vi "SetNeoParams.vi"(4 "Error In":errorcluster, 5 "Debug":bool=TRUE) -> (0 "ErrorOut":errorcluster, 3 "Handle":i32)   [LabVIEW 2014]
panel:
  in  "PreAmp Gain Control":string(combo)="16-bit (low noise & high well capacity)"
  out "Stat: preamp":i32
  in  "Cluster":T1={"ExposureTime"=0.1, "AOI Height"=2160, "AOI Width"=2560}
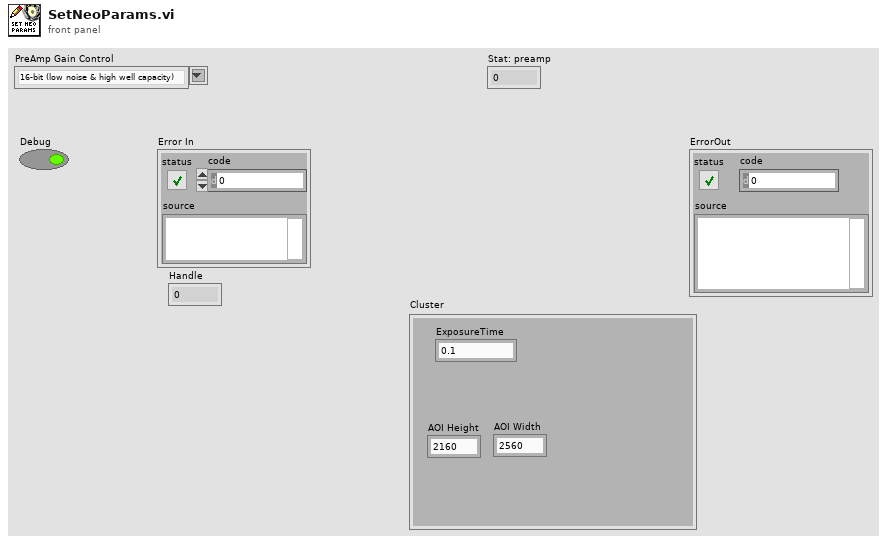
[diagram p1: front panel]
types:
  T1 = cluster{"ExposureTime":dbl, "AOI Height":i32, "AOI Width":i32}
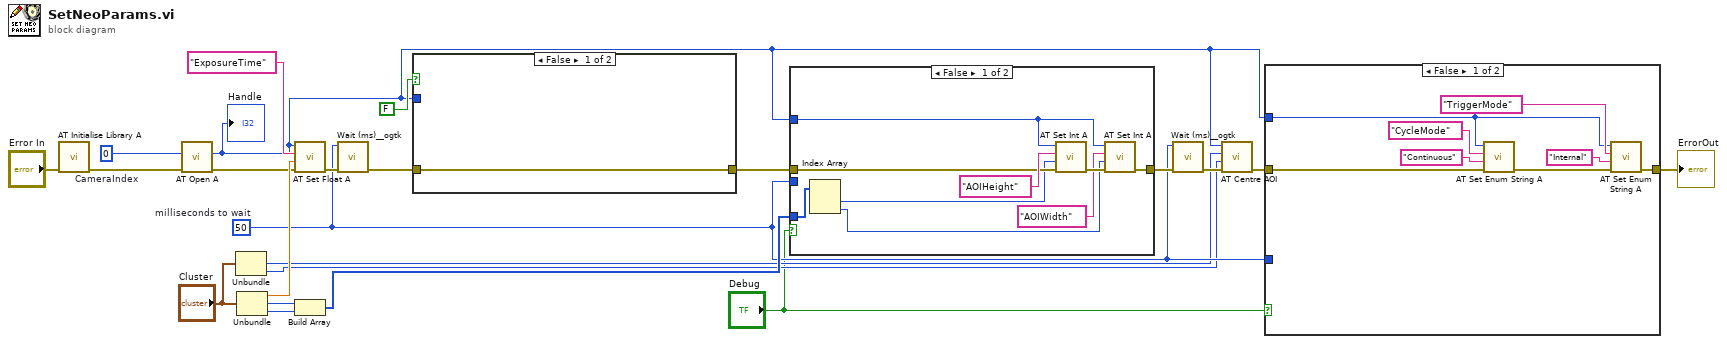
[diagram p0: block diagram]
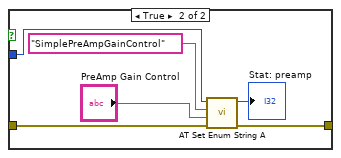
[diagram p2: hidden frame]
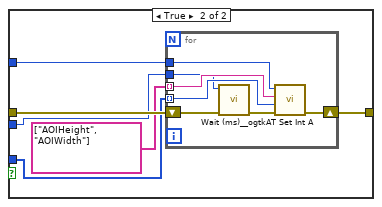
[diagram p3: hidden frame]
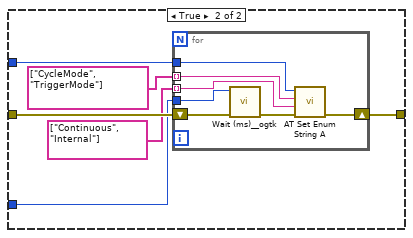
[diagram p4: hidden frame]
diagram:
  w4 = 0  # CameraIndex
  w13 = u32 50  # milliseconds to wait
  n1 = call <userlib>:"AT Initialise Library A.vi"("error in (no error)"="Error In") -> ("error out"=w5:errorcluster)  [unwired: 9 in, 1 out]
  n2 = call <userlib>:"AT Open A.vi"("error in (no error)"=w5, "CameraIndex"=w4) -> ("error out"=w3:errorcluster, "Handle"=w1:i32)  [unwired: 7 in, 1 out]
  "Handle" <- w1
  n3 = Unbundle("Cluster") -> ("AOI Height"=w10:i32, "AOI Width"=w9:i32)  [unwired: 1 out]
  n4 = Unbundle("Cluster") -> ("ExposureTime"=w20:dbl, "AOI Height"=w12:i32, "AOI Width"=w11:i32)
  n5 = call <userlib>:"AT Set Float A.vi"("error in (no error)"=w3, "Value"=w20, "Feature"="ExposureTime" ("ExposureTime"), "Hndl"=w1) -> ("error out"=w22:errorcluster)  [unwired: 6 in, 1 out]
  n6 = Build Array(w12, w11) -> (w19:i32[])
  n7 = call <userlib>:"Wait (ms)__ogtk.vi"("error in (no error)"=w22, "milliseconds to wait"=w13) -> ("error out"=w8:errorcluster)  [unwired: 8 in, 1 out]
  n8 = case shown="False" FALSE {
    tunnel: [w24 w29] -> w21
    tunnel: w1 -> [_ w28]
    tunnel: w8 -> [w24 w25]
    frame False {
    }
    frame True {
      n9 = call <userlib>:"AT Set Enum String A.vi"("error in (no error)"=w25, "String"="PreAmp Gain Control", "Feature"="SimplePreAmpGainControl" ("Enum feature"), "Handle"=w28) -> ("error out"=w29:errorcluster, "Status"=→"Stat: preamp":i32)  [unwired: 6 in]
    }
  }
  n10 = case shown="False" "Debug" {
    tunnel: w21 -> [w34 w45]
    tunnel: w19 -> [w39 w43]
    tunnel: w1 -> [w33 w42]
    tunnel: [w35 w41] -> w15
    tunnel: w13 -> [_ w40]
    frame False {
      n11 = Index Array(array=w39) -> (element #1=w32:i32, element #2=w31:i32)  [unwired: 2 in]
      n12 = call <userlib>:"AT Set Int A.vi"("error in (no error)"=w34, "Value"=w32, "Feature"="AOIHeight" ("Integer feature"), "Handle"=w33) -> ("error out"=w38:errorcluster)  [unwired: 6 in, 1 out]
      n13 = call <userlib>:"AT Set Int A.vi"("error in (no error)"=w38, "Value"=w31, "Feature"="AOIWidth" ("Integer feature 2"), "Handle"=w33) -> ("error out"=w35:errorcluster)  [unwired: 6 in, 1 out]
    }
    frame True {
      n14 = for {
        tunnel: string[] ["AOIHeight", "AOIWidth"] -> [w52] mode=indexing
        tunnel: w42 -> [w51]
        shift-right: [w50] -> w41
        shift-left: w45 -> [w49]
        tunnel: w43 -> [w47] mode=indexing
        tunnel: w40 -> [w46]
        n15 = call <userlib>:"Wait (ms)__ogtk.vi"("error in (no error)"=w49, "milliseconds to wait"=w46) -> ("error out"=w48:errorcluster)  [unwired: 8 in, 1 out]
        n16 = call <userlib>:"AT Set Int A.vi"("error in (no error)"=w48, "Value"=w47, "Feature"=w52, "Handle"=w51) -> ("error out"=w50:errorcluster)  [unwired: 6 in, 1 out]
      }
    }
  }
  n17 = call <userlib>:"Wait (ms)__ogtk.vi"("error in (no error)"=w15, "milliseconds to wait"=w13) -> ("error out"=w14:errorcluster)  [unwired: 8 in, 1 out]
  n18 = call <userlib>:"AT Centre AOI.vi"("error in (no error)"=w14, "AOI Width"=w9, "AOI Height"=w10, "Handle"=w1) -> ("error out"=w17:errorcluster)  [unwired: 7 in]
  n19 = case shown="False" "Debug" {
    tunnel: w1 -> [w55 w66]
    tunnel: w17 -> [w53 w65]
    tunnel: [w58 w64] -> w16
    tunnel: w13 -> [_ w61]
    frame False {
      n20 = call <userlib>:"AT Set Enum String A.vi"("error in (no error)"=w53, "String"="Continuous", "Feature"="CycleMode" ("Enum feature"), "Handle"=w55) -> ("error out"=w54:errorcluster)  [unwired: 6 in, 1 out]
      n21 = call <userlib>:"AT Set Enum String A.vi"("error in (no error)"=w54, "String"="Internal", "Feature"="TriggerMode" ("Enum feature"), "Handle"=w55) -> ("error out"=w58:errorcluster)  [unwired: 6 in, 1 out]
    }
    frame True {
      n22 = for {
        tunnel: string[] ["Continuous", "Internal"] -> [w73] mode=indexing
        tunnel: string[] ["CycleMode", "TriggerMode"] -> [w72] mode=indexing
        tunnel: w66 -> [w71]
        shift-right: [w70] -> w64
        shift-left: w65 -> [w69]
        tunnel: w61 -> [w67]
        n23 = call <userlib>:"Wait (ms)__ogtk.vi"("error in (no error)"=w69, "milliseconds to wait"=w67) -> ("error out"=w68:errorcluster)  [unwired: 8 in, 1 out]
        n24 = call <userlib>:"AT Set Enum String A.vi"("error in (no error)"=w68, "String"=w73, "Feature"=w72, "Handle"=w71) -> ("error out"=w70:errorcluster)  [unwired: 6 in, 1 out]
      }
    }
  }
  "ErrorOut" <- w16
